vi "AutoDriveDistance.vi"(6 "StartTime(ms)":u32, 7 "TurnSpeed":dbl, 8 "MaxRampRate(%/s)":dbl, 9 "MaxSpeed":dbl, 10 "Distance(in)":dbl, 11 "StartDistance":dbl) -> (3 "Complete":bool)   [LabVIEW 2019]
uses:
  Global_Var-RefNum/RobotState.vi
  Global_Var-RefNum/AutoCommands.vi
  ArgosLib/ArgosLib.lvlib
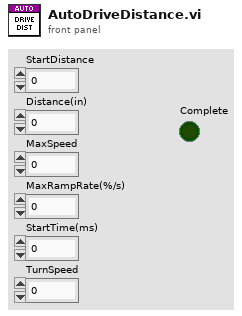
[diagram p1: front panel]
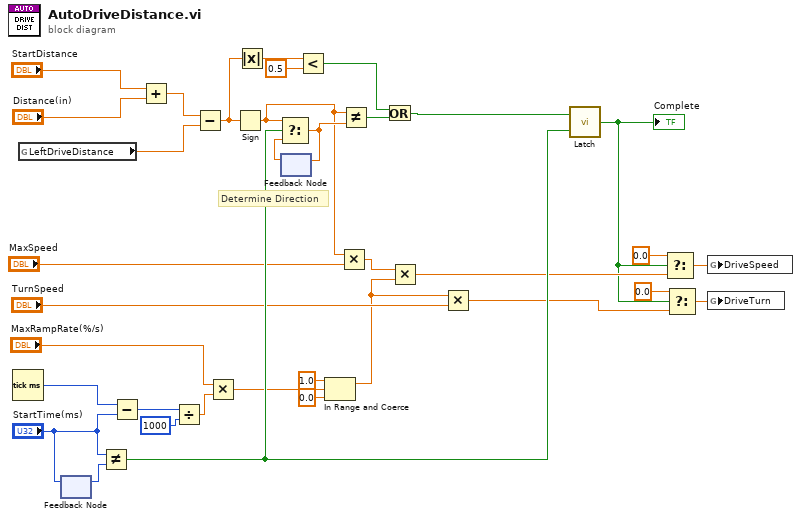
[diagram p0: block diagram]
diagram:
  # "Determine Direction"
  n1 = Tick Count (ms)() -> (millisecond timer value=w35:u32)
  n2 = global read "RobotState.vi" "LeftDriveDistance"() -> (w29:dbl)
  n3 = feedback-in #1("StartTime(ms)") -> ()
  n4 = feedback #1() -> (w32:u32)  [unwired: 1 in]
  n5 = Not Equal?(x="StartTime(ms)", y=w32) -> (x != y?=w27:bool)
  n6 = Subtract(x=w35, y="StartTime(ms)") -> (x-y=w17:u32)
  n7 = Add(x="StartDistance", y="Distance(in)") -> (x+y=w30:dbl)
  n8 = Divide(x=w17, y=u32 1000) -> (x/y=w15:dbl)
  n9 = Subtract(x=w30, y=w29) -> (x-y=w24:dbl)
  n10 = Multiply(x="MaxRampRate(%/s)", y=w15) -> (x*y=w13:dbl)
  n11 = Sign(1:w24) -> (0:w19:dbl)
  n12 = Absolute Value(x=w24) -> (abs(x)=w23:dbl)
  n13 = feedback #2() -> (w28:dbl)  [unwired: 1 in]
  n14 = Select(t=w19, s=w27, f=w28) -> (s? t:f=w26:dbl)
  n15 = feedback-in #2(w26) -> ()
  n16 = Less?(x=w23, y=0.5) -> (x < y?=w21:bool)
  n17 = In Range and Coerce(upper limit=1.0, x=w13, lower limit=0.0) -> (coerced(x)=w5:dbl)  [unwired: 1 out]
  n18 = Multiply(x=w19, y="MaxSpeed") -> (x*y=w10:dbl)
  n19 = Not Equal?(x=w19, y=w26) -> (x != y?=w25:bool)
  n20 = Or(x=w21, y=w25) -> (x .or. y?=w20:bool)
  n21 = Multiply(x=w10, y=w5) -> (x*y=w7:dbl)
  n22 = Multiply(x=w5, y="TurnSpeed") -> (x*y=w3:dbl)
  n23 = call "Latch.vi"("Reset"=w27, "Input"=w20) -> ("LatchOut"=w1:bool)
  "Complete" <- w1
  n24 = Select(t=0.0, s=w1, f=w7) -> (s? t:f=w9:dbl)
  n25 = Select(t=0.0, s=w1, f=w3) -> (s? t:f=w2:dbl)
  n26 = global write "AutoCommands.vi" "DriveSpeed"(w9) -> ()
  n27 = global write "AutoCommands.vi" "DriveTurn"(w2) -> ()
